vi "FPGA_target_find_stop_output.vi"(5 "start_addr":u32, 7 "number_cmds_in":u32) -> (10 "found":bool, 11 "C1_data":T1, 13 "number_cmds_dup":u32)   [LabVIEW 2014]
doc: "This VI searchs the next stop command following the start address."
uses:
  FPGA_32BitPattern_data_type.ctl
  <vilib>/rvi/Emulation/niFpgaCriticalErrorInLSC.vi
  <vilib>/rvi/Emulation/niFpgaEmulationReportErrorSimple.vi
  <vilib>/rvi/Emulation/niFpgaSctlEmulationGetInTimedLoop.vi
  <vilib>/rvi/Emulation/niFpgaGetClockAttributes.vi
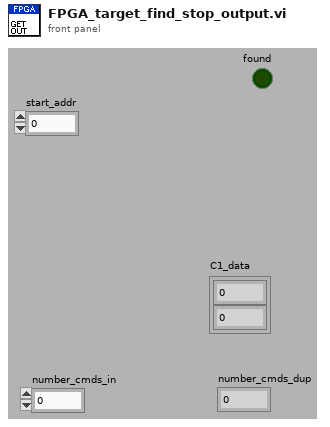
[diagram p1: front panel]
types:
  T1 = typedef "FPGA_32BitPattern_data_type.ctl" = cluster{"port0":u8, "port1":u8}
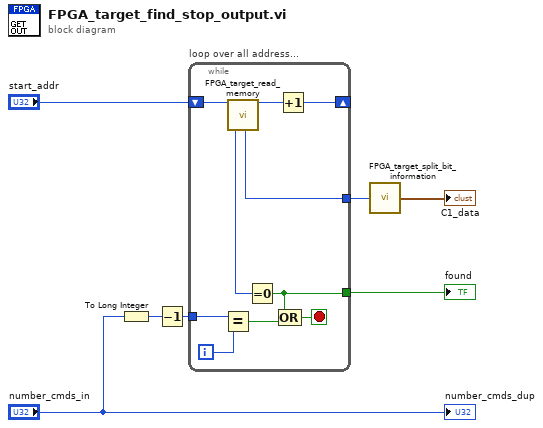
[diagram p0: block diagram]
diagram:
  n1 = To Long Integer(number="number_cmds_in") -> (32bit integer=w5:i32)
  n2 = Decrement(x=w5) -> (x-1=w6:i32)
  n3 = while "loop over all address..." {
    tunnel: w6 -> [w13]
    shift-right: [w11] -> _
    shift-left: "start_addr" -> [w17]
    tunnel: [w9] -> w4
    tunnel: [w8] -> w2
    i -> [w15]
    stop <- w10 stop-if-true
    n4 = Equal?(x=w13, y=w15) -> (x = y?=w12:bool)
    n5 = call "FPGA_target_read_memory.vi"("addr_in"=w17) -> ("data_mem0"=w16:u8, "data_mem2"=w9:u16, "addr_dup"=w14:u32)  [unwired: 14 in, 2 out]
    n6 = Equal To 0?(x=w16) -> (x = 0?=w8:bool)
    n7 = Increment(x=w14) -> (x+1=w11:u32)
    n8 = Compound Arithmetic op=OR(w8, w12) -> (w10:bool)
  }
  "found" <- w2
  n9 = call "FPGA_target_split_bit_information.vi"("data in"=w4) -> ("connector_data"=→"C1_data":T1)
  "number_cmds_dup" <- "number_cmds_in"
